vi "Check Status.vi"(7 "VI Action":T1=enum."Write", 8 "Index":i32, 9 "Tolerance":dbl=10.0, 10 "Value Read":dbl, 11 "Value Set":dbl) -> (3 "Array":bool[](array[boolean]))   [LabVIEW 2010]
uses:
  status action.ctl
panel:
  out "Status":bool
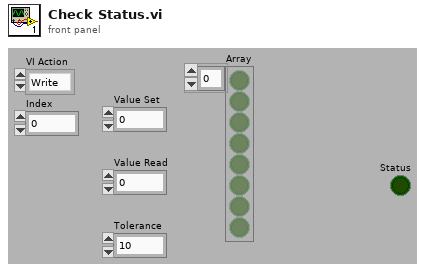
[diagram p1: front panel]
types:
  T1 = typedef "status action.ctl" = enum16{"Initialize", "Write", "Read"}
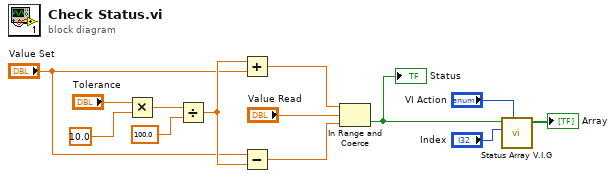
[diagram p0: block diagram]
diagram:
  n1 = Multiply(x="Tolerance", y=10.0) -> (x*y=w10:dbl)
  n2 = Divide(x=w10, y=100.0) -> (x/y=w13:dbl)
  n3 = Add(x=w13, y="Value Set") -> (x+y=w6:dbl)
  n4 = Subtract(x="Value Set", y=w13) -> (x-y=w7:dbl)
  n5 = In Range and Coerce(upper limit=w6, x="Value Read", lower limit=w7) -> (In Range?=w1:bool)  [unwired: 1 out]
  "Status" <- w1
  n6 = call "Status Array V.I.G.vi"("VI Action"="VI Action", "index"="Index", "Element"=w1) -> ("Array"=→"Array":bool[])  [unwired: 8 in]
